vi "AddToProcessorEnqueuerList.vi"(8 "error in (no error)":errorcluster, 9 "Label":string, 10 "ProcessorEnqueuer":refnum<class "Message Enqueuer.lvclass">, 11 "Microscope in":refnum<class "Microscope.lvclass">) -> (0 "error out":errorcluster, 1 "value unchanged?":bool, 2 "key already included?":bool, 3 "Microscope out":refnum<class "Microscope.lvclass">)   [LabVIEW 2020, in "Microscope.lvlib" / "Microscope.lvclass"]
uses:
  Microscope.lvclass
  <vilib>/ActorFramework/Message Enqueuer/Message Enqueuer.lvclass
  Microscope.lvclass/Microscope.ctl
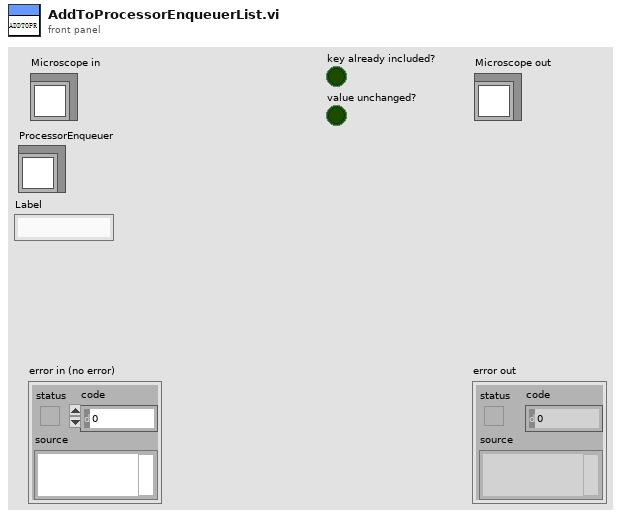
[diagram p1: front panel]
types:
  T1 = map{string, refnum<class "Message Enqueuer.lvclass">}
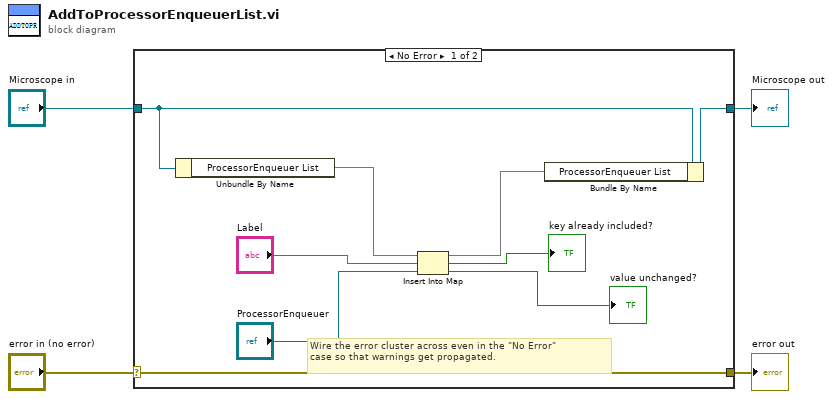
[diagram p0: block diagram]
diagram:
  n1 = case shown="No Error" "error in (no error)" {
    selector: "error in (no error)" -> [w13 w15]
    tunnel: [w13 w15] -> w3
    tunnel: [w11 w14] -> w1
    tunnel: "Microscope in" -> [w12 w14]
    frame No Error {
      # "Wire the error cluster across even in the \"No Error\"\ncase so that warnings get propagated."
      n2 = Unbundle By Name(w12) -> ("ProcessorEnqueuer List"=w10:T1)
      n3 = Insert Into Map(map in=w10, key="Label", value="ProcessorEnqueuer") -> (map out=w9:T1, key already included?=→"key already included?":bool, value unchanged?=→"value unchanged?":bool)
      n4 = Bundle By Name(cluster=w12, "ProcessorEnqueuer List"=w9) -> (w11:refnum<class "Microscope.lvclass">)
    }
    frame Error {
    }
  }
  "error out" <- w3
  "Microscope out" <- w1
